vi "Counter.vi"(9 "Photo Eye 0":bool, 10 "Button 0":bool) -> (1 "Ball Count":i32)   [LabVIEW 2019]
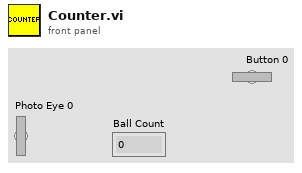
[diagram p1: front panel]
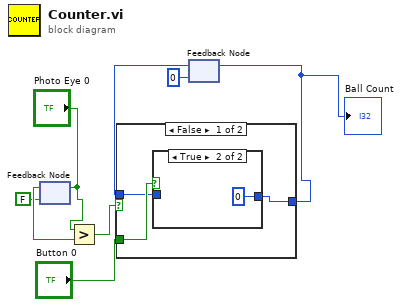
[diagram p0: block diagram]
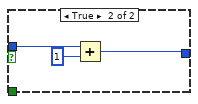
[diagram p3: hidden frame]
diagram:
  n1 = feedback #1(FALSE ("Boolean")) -> (w7:bool)
  n2 = feedback-in #1("Photo Eye 0") -> ()
  n3 = Greater?(x="Photo Eye 0", y=w7) -> (0:w5:bool)
  n4 = feedback #2(0) -> (w8:i32)
  n5 = case shown="False" w5 {
    tunnel: [w10 w16] -> w2
    tunnel: w8 -> [w9 w15]
    tunnel: "Button 0" -> [w11 _]
    frame False {
      n6 = case shown="True" w11 {
        tunnel: [w12 0] -> w10
        tunnel: w9 -> [w12 _]
        frame False {
        }
        frame True {
        }
      }
    }
    frame True {
      n7 = Add(x=w15, y=1) -> (x+y=w16:i32)
    }
  }
  "Ball Count" <- w2
  n8 = feedback-in #2(w2) -> ()
